vi "RTP_Bus_v2.vi"() -> ()   [LabVIEW 2015]
uses:
  <vilib>/myRIO/Common/Instrument Driver Framework/myRIO v1.0/UART/vis/myRIO v1.0 Close UART.vi
  <vilib>/FPGAPlugInAG/myRIO-1900/niLvFpga_Open_myRIO-1900.vi
  <vilib>/rvi/interface/common/dynamic/niFpgaDynamicAddResources.vi
  <vilib>/Utility/error.llb/Error Cluster From Error Code.vi
  <vilib>/rvi/errors/niLvFpgaAdjustHostInterfaceError.vi
  <vilib>/FPGAPlugInAG/Dynamic/niLvFpga_Close_Dynamic.vi
  <vilib>/myRIO/Common/Instrument Driver Framework/Utilities/vis/FPGA Ref Manager.vi
  <vilib>/myRIO/Common/Instrument Driver Framework/myRIO v1.0/myRIO v1.0 Reset FPGA.vi
  <vilib>/myRIO/Common/Instrument Driver Framework/myRIO v1.0/IRQ/vis/myRIO v1.0 IRQ Info FGV.vi
  <vilib>/myRIO/Common/Instrument Driver Framework/myRIO v1.0/IRQ/vis/myRIO v1.0 Timer IRQ Info FGV.vi
  <vilib>/myRIO/Common/Instrument Driver Framework/myRIO v1.0/IRQ/vis/myRIO v1.0 ISR Agent.vi
  <vilib>/rvi/interface/nirviOpenFPGA/nirviOpenFPGA.xnode
  FPGA Bitfiles/CurShar_FPGATarget2_FPGABus_q7Z4AXA+lvw.lvbitx
  FPGA_Bus.vi
  <vilib>/rvi/interface/nirviReadWriteControl/nirviReadWriteControl.xnode
  <vilib>/rvi/interface/nirviCloseFPGA/nirviCloseFPGA.xnode
  <vilib>/myRIO/Instrument Drivers/Utilities/Utilities.lvlib
  NiFpgaLv.dll
  <vilib>/rvi/interface/Simulation/niFpgaSimulationCallBeginRW.vi
panel:
  out "T":u32
  in  "stop":bool
  out "activ":cluster{dbl[], i16[]}[](graph)
  out "T":u32
  out "R":cluster{dbl[], dbl[]}(graph)
  out "e3":cluster{dbl[], i16[]}(graph)
  out "e2":cluster{dbl[], i16[]}(graph)
  out "e1":cluster{dbl[], i16[]}(graph)
  in  "start":bool
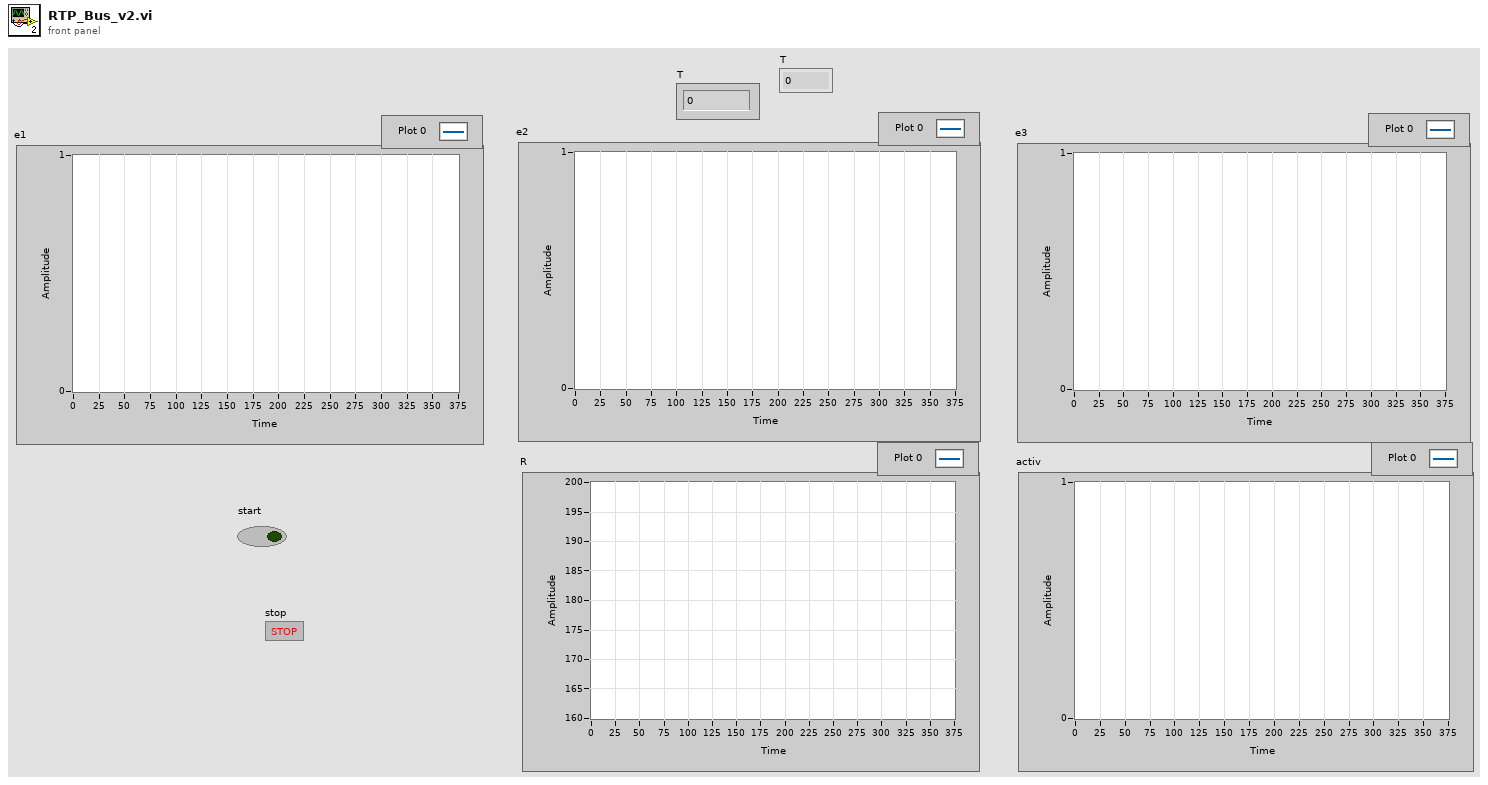
[diagram p1: front panel]
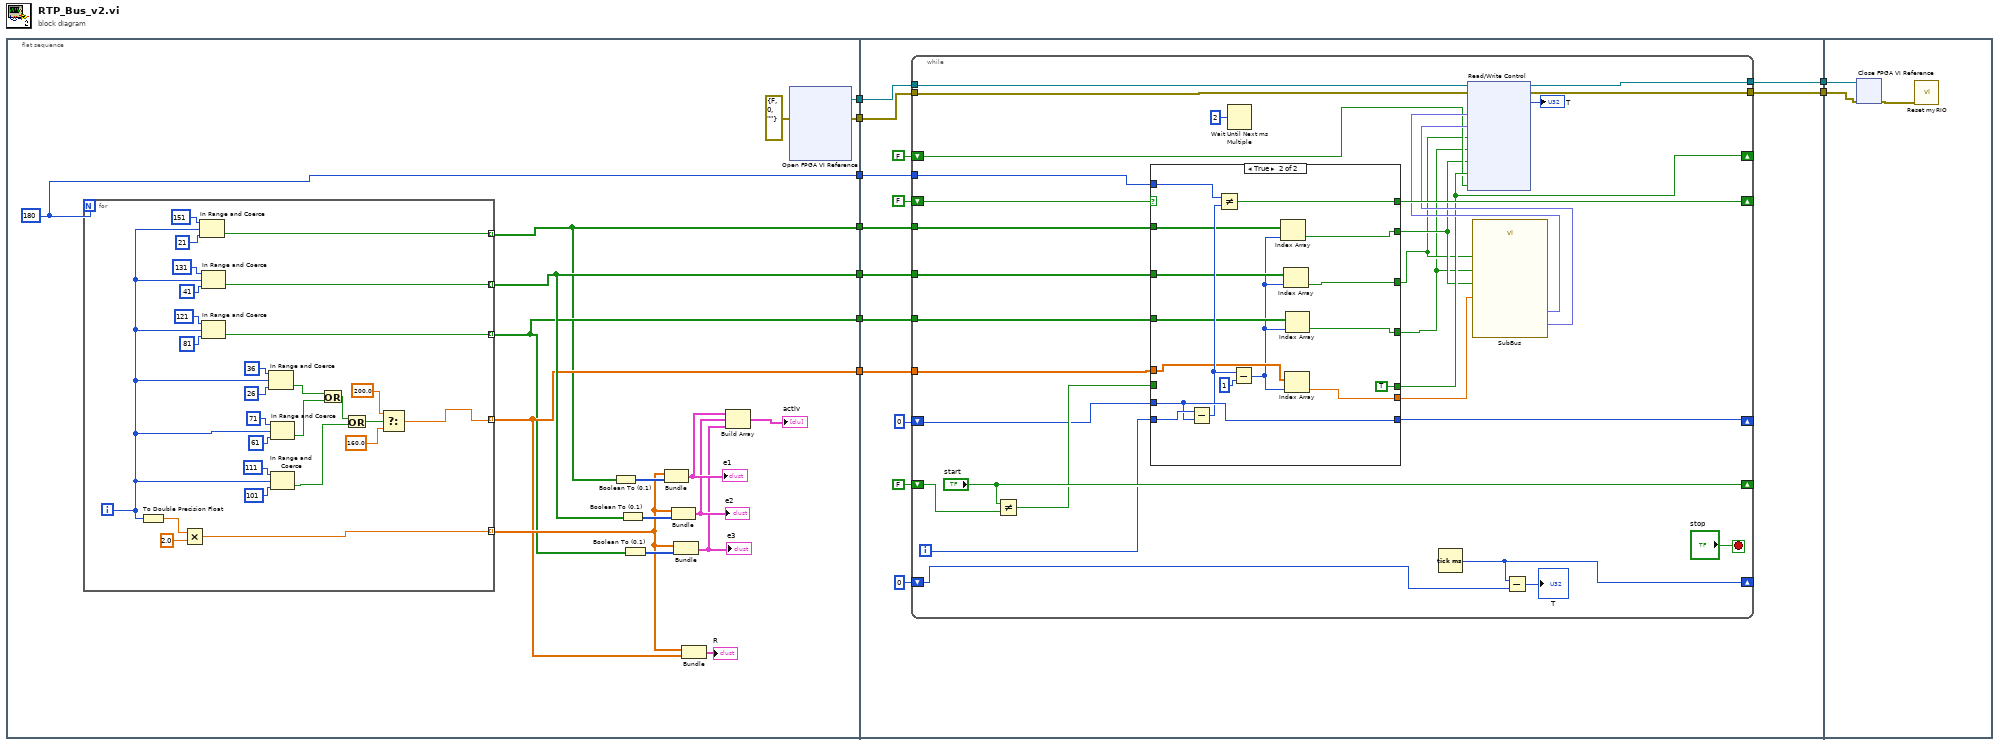
[diagram p0: block diagram]
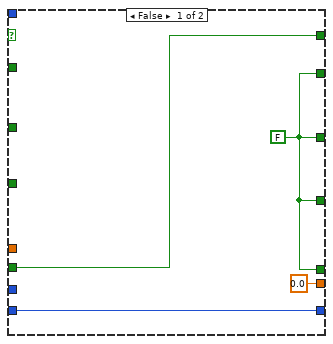
[diagram p2: hidden frame]
diagram:
  n1 = flat-sequence {
    tunnel: [w25] -> w9
    tunnel: [w24] -> w8
    tunnel: [w10] -> w7
    tunnel: [w20] -> w6
    tunnel: [w11] -> w5
    tunnel: [w17] -> w4
    tunnel: [w12] -> w3
    tunnel: w9 -> [w64]
    tunnel: w8 -> [w63]
    tunnel: w7 -> [w62]
    tunnel: w6 -> [w61]
    tunnel: w5 -> [w60]
    tunnel: w4 -> [w59]
    tunnel: w3 -> [w58]
    tunnel: [w57] -> w2
    tunnel: [w56] -> w1
    tunnel: w2 -> [w121]
    tunnel: w1 -> [w120]
    frame #0 {
      w12 = 180
      n2 = for {
        N: w12 -> [_]
        tunnel: [w47] -> w10 mode=indexing
        tunnel: [w46] -> w20 mode=indexing
        tunnel: [w45] -> w11 mode=indexing
        tunnel: [w27] -> w17 mode=indexing
        tunnel: [w42] -> w18 mode=indexing
        i -> [w35]
        n3 = To Double Precision Float(number=w35) -> (double precision float=w44:dbl)
        n4 = Multiply(x=w44, y=2.0) -> (x*y=w42:dbl)
        n5 = In Range and Coerce(upper limit=151, x=w35, lower limit=21) -> (In Range?=w47:bool)  [unwired: 1 out]
        n6 = In Range and Coerce(upper limit=131, x=w35, lower limit=41) -> (In Range?=w46:bool)  [unwired: 1 out]
        n7 = In Range and Coerce(upper limit=121, x=w35, lower limit=81) -> (In Range?=w45:bool)  [unwired: 1 out]
        n8 = In Range and Coerce(upper limit=36, x=w35, lower limit=26) -> (In Range?=w34:bool)  [unwired: 1 out]
        n9 = In Range and Coerce(upper limit=71, x=w35, lower limit=61) -> (In Range?=w33:bool)  [unwired: 1 out]
        n10 = In Range and Coerce(upper limit=111, x=w35, lower limit=101) -> (In Range?=w31:bool)  [unwired: 1 out]
        n11 = Or(x=w34, y=w33) -> (x .or. y?=w32:bool)
        n12 = Or(x=w32, y=w31) -> (x .or. y?=w30:bool)
        n13 = Select(t=200.0, s=w30, f=160.0) -> (s? t:f=w27:dbl)
      }
      n14 = Boolean To (0,1)(Boolean=w10) -> (0, 1=w23:i16[])
      n15 = Boolean To (0,1)(Boolean=w20) -> (0, 1=w22:i16[])
      n16 = Boolean To (0,1)(Boolean=w11) -> (0, 1=w21:i16[])
      n17 = Bundle(w18, w23) -> (w16:cluster{dbl[], i16[]})  [unwired: 1 in]
      "e1" <- w16
      n18 = Bundle(w18, w22) -> (w15:cluster{dbl[], i16[]})  [unwired: 1 in]
      "e2" <- w15
      n19 = Bundle(w18, w21) -> (w14:cluster{dbl[], i16[]})  [unwired: 1 in]
      "e3" <- w14
      n20 = Bundle(w18, w17) -> (→"R":cluster{dbl[], dbl[]})  [unwired: 1 in]
      n21 = Build Array(w16, w15, w14) -> (→"activ":cluster{dbl[], i16[]}[])
      n22 = xnode "Open FPGA VI Reference"("error in"=errorcluster {"status"=FALSE, "code"=0, "source"=""}) -> ("FPGA VI Reference Out"=w25:refnum<k20>, "error out"=w24:errorcluster)  [unwired: 1 in]
    }
    frame #1 {
      n23 = while {
        shift-right: ["start"] -> _
        shift-left: FALSE ("start") -> [w97]
        shift-right: [w95] -> _
        shift-left: FALSE -> [w96]
        shift-right: [w93] -> _
        shift-left: 0 -> [w91]
        tunnel: w64 -> [w90]
        tunnel: w63 -> [w89]
        tunnel: w62 -> [w86]
        tunnel: w61 -> [w85]
        tunnel: w60 -> [w84]
        tunnel: w59 -> [w83]
        tunnel: w58 -> [w81]
        tunnel: [w80] -> w57
        tunnel: [w79] -> w56
        shift-right: [w75] -> _
        shift-left: u32 0 ("millisecond timer value") -> [w74]
        shift-right: [w72] -> _
        shift-left: FALSE -> [w71]
        i -> [w92]
        stop <- "stop" stop-if-true
        n24 = Not Equal?(x="start", y=w97) -> (x != y?=w94:bool)
        n25 = case shown="True" w96 {
          tunnel: [w102 w116] -> w95
          tunnel: w94 -> [w102 _]
          tunnel: [w101 w117] -> w93
          tunnel: w92 -> [w101 w118]
          tunnel: w91 -> [_ w117]
          tunnel: [w100 w110] -> w70
          tunnel: [w100 w109] -> w69
          tunnel: [w100 w108] -> w68
          tunnel: [w100 TRUE] -> w72
          tunnel: w86 -> [_ w113]
          tunnel: w85 -> [_ w112]
          tunnel: w84 -> [_ w111]
          tunnel: w83 -> [_ w107]
          tunnel: [0.0 w105] -> w82
          tunnel: w81 -> [_ w104]
          frame False {
            w100 = FALSE
          }
          frame True {
            n26 = Subtract(x=w118, y=w117) -> (x-y=w115:i32)
            n27 = Not Equal?(x=w104, y=w115) -> (x != y?=w116:bool)
            n28 = Subtract(x=w115, y=1) -> (x-y=w106:i32)
            n29 = Index Array(array=w113, index=w106) -> (element=w110:bool)
            n30 = Index Array(array=w112, index=w106) -> (element=w109:bool)
            n31 = Index Array(array=w107, index=w106) -> (element=w105:dbl)
            n32 = Index Array(array=w111, index=w106) -> (element=w108:bool)
          }
        }
        n33 = Wait Until Next ms Multiple(millisecond multiple=u32 2) -> ()  [unwired: 1 out]
        n34 = Tick Count (ms)() -> (millisecond timer value=w75:u32)
        n35 = call "SubBus.vi"("R"=w82, "e3"=w70, "e2"=w68, "e1"=w69) -> ("1-T/(R*e*C)"=w88:fxp<+,20,0>, "T/(e*C)"=w87:fxp<+,20,0>)  [unwired: 6 in]
        n36 = xnode "Read/Write Control"("FPGA VI Reference In"=w90, "error in"=w89, "1-T/(R*e*C)"=w88, "T/(e*C)"=w87, "e1"=w69, "e2"=w68, "e3"=w70, "trigger"=w72, "start"=w71) -> ("FPGA VI Reference Out"=w80:refnum<k20>, "error out"=w79:errorcluster, "T"=→"T":u32)
        n37 = Subtract(x=w75, y=w74) -> (x-y=→"T":u32)
      }
    }
    frame #2 {
      n38 = xnode "Close FPGA VI Reference"("FPGA VI Reference In"=w121, "error in"=w120) -> ("error out"=w119:errorcluster)
      n39 = call <vilib>:"Reset myRIO.vi"("error in (no error)"=w119) -> ()  [unwired: 10 in, 1 out]
    }
  }
